vi "Global visibility tickbox-Groups.vi"(8 "error in (no error)":errorcluster) -> (0 "error out":errorcluster)   [LabVIEW 2020]
uses:
  Global variables/gl_Functional Imaging-Global variables.vi
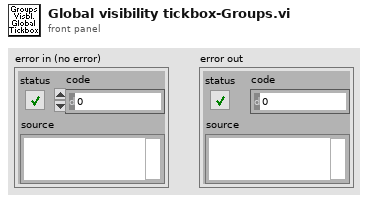
[diagram p1: front panel]
types:
  T1 = typedef "Functional Imging UI Refs.ctl" = cluster{"Menu ref":refnum<k9>, "Image control":refnum<vi>, "VI ref":refnum<vi>, "XGrapher":refnum<vi>, "Smoothing":refnum<vi>, "POI Averaging":refnum<vi>, "Normalize":refnum<vi>, "POI data points in each trial":refnum<vi>, "Channel":refnum<vi>, "Experiment data folder path":refnum<vi>, "[ROI vis]":refnum<vi>, "[Groups] visbl":T2, "Group Name":refnum<vi>, "POI index":refnum<vi>, "Trial No.":refnum<vi>, "Intensity Zoom":refnum<vi>, "Trial Cursor Enabled":refnum<vi>, "Number of Trials (ind 1)":refnum<vi>, "Number of Trials (ind 2)":refnum<vi>, "MiniScans Available":refnum<vi>, "POI Available":refnum<vi>, "Defer graph updates":refnum<vi>, "Waveform selector":refnum<vi>, "#of selected POI":refnum<vi>, "#of selected MiniScans":refnum<vi>, "#of selected groups":refnum<vi>, "Max Z-Projection":refnum<vi>, "Z-Plane Selector":refnum<vi>, "Index of miniscan point to visualise":refnum<vi>, "ROI vis. mode":refnum<vi>, "Total # of points":refnum<vi>, "Index of group clicked on":refnum<vi>, "Pane 1":refnum<vi>, "Pane 2":refnum<vi>, "Pane 3":refnum<vi>, "Pane 4":refnum<vi>, "Pane 5":refnum<vi>, "Pane 6":refnum<vi>, "Deselect all ROI":refnum<vi>, "Deselect all groups":refnum<vi>}
  T2 = typedef "Groups array referecne.ctl" = refnum<vi>
  T3 = typedef "Group sel cluster.ctl" = cluster{"Group number":string, "Group Name":string, "Visibility":bool, "Highlight":bool}
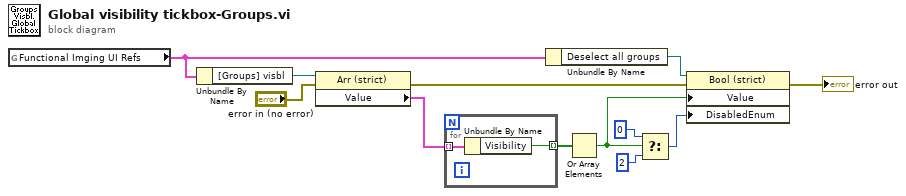
[diagram p0: block diagram]
diagram:
  n1 = global read "gl_Functional Imaging-Global variables.vi" "Functional Imging UI Refs"() -> (w6:T1)
  n2 = Unbundle By Name(w6) -> ("[Groups] visbl"=w5:T2)
  n3 = property on="Property Node" class="Arr (strict)"(reference=w5, error in="error in (no error)") -> (error out=w7:errorcluster, "Value"=w3:T3[])  [unwired: 1 out]
  n4 = for {
    tunnel: w3 -> [w14] mode=indexing
    tunnel: [w13] -> w4 mode=indexing
    n5 = Unbundle By Name(w14) -> ("Visibility"=w13:bool)
  }
  n6 = Unbundle By Name(w6) -> ("Deselect all groups"=w1:refnum<vi>)
  n7 = Or Array Elements(Boolean array=w4) -> (logical OR=w9:bool)
  n8 = Select(t=0, s=w9, f=2) -> (s? t:f=w12:i32)
  n9 = property on="Property Node" class="Bool (strict)"(reference=w1, error in=w7, "Value"=w9, "DisabledEnum"=w12) -> (error out=→"error out":errorcluster)  [unwired: 1 out]
